vi "IO.vi"(8 "error in (no error)":errorcluster caption="错误输入（无错误）", 10 "write":string, 11 "VISA resource name":refnum<visa-resource-name> caption="VISA资源名称") -> (0 "错误输出":errorcluster, 3 "read":string)   [LabVIEW 2018, in "qingshan.lvlib"]
uses:
  qingshan.lvlib
  <vilib>/Instr/_visa.llb/VISA Configure Serial Port (Instr).vi
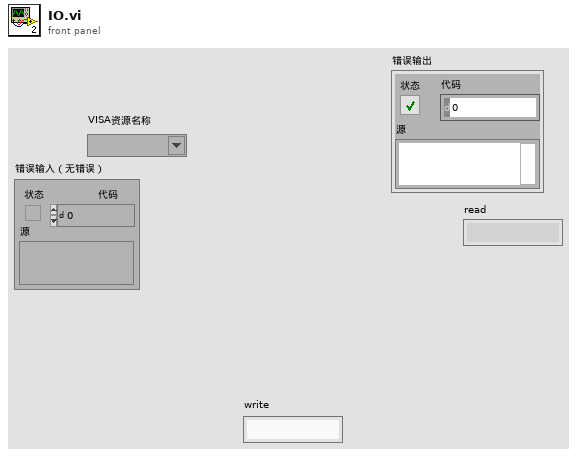
[diagram p1: front panel]
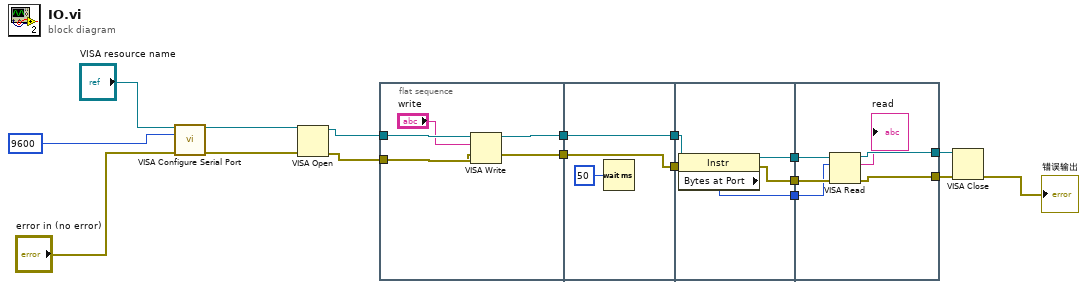
[diagram p0: block diagram]
diagram:
  n1 = call-poly "VISA Configure Serial Port"("VISA resource name"="VISA resource name", "baud rate (9600)"=u32 9600, "error in (no error)"="error in (no error)") -> ("VISA resource name out"=w17:refnum<visa-resource-name>, "error out"=w16:errorcluster)  [unwired: 11 in]
  n2 = VISA Open(error in (no error)=w16, VISA resource name=w17) -> (VISA resource name=w15:refnum<visa-resource-name>, error out=w14:errorcluster)  [unwired: 3 in]
  n3 = flat-sequence {
    tunnel: w15 -> [w22]
    tunnel: w14 -> [w21]
    tunnel: [w20] -> w12
    tunnel: [w19] -> w10
    tunnel: [w24] -> w13
    tunnel: w12 -> [w24]
    tunnel: [w23] -> w11
    tunnel: w10 -> [w23]
    tunnel: w13 -> [w30]
    tunnel: w11 -> [w29]
    tunnel: [w28] -> w9
    tunnel: [w27] -> w8
    tunnel: [w26] -> w3
    tunnel: w9 -> [w36]
    tunnel: w8 -> [w35]
    tunnel: [w34] -> w7
    tunnel: [w33] -> w6
    tunnel: w3 -> [w31]
    frame #0 {
      n4 = VISA Write(VISA resource name=w22, write buffer="write", error in (no error)=w21) -> (VISA resource name out=w20:refnum<visa-resource-name>, error out=w19:errorcluster)  [unwired: 1 out]
    }
    frame #1 {
      n5 = Wait (ms)(milliseconds to wait=u32 50 ("等待时间（毫秒）")) -> ()  [unwired: 1 out]
    }
    frame #2 {
      n6 = property class="Instr"(reference=w30, error in=w29) -> (reference out=w28:refnum<visa-resource-name>, error out=w27:errorcluster, "Bytes at Port"=w26:u32)
    }
    frame #3 {
      n7 = VISA Read(VISA resource name=w36, byte count=w31, error in (no error)=w35) -> (VISA resource name out=w34:refnum<visa-resource-name>, read buffer=→"read":string, error out=w33:errorcluster)  [unwired: 1 out]
    }
  }
  n8 = VISA Close(VISA resource name=w7, error in (no error)=w6) -> (error out=→"错误输出":errorcluster)
